vi "Global_SEN_Data Out.vi"() -> ()   [LabVIEW 2020, in "GameController_SEN.lvlib"]
uses:
  GameController_SEN.lvlib
panel:
  in  "SEN_GameController_POVs 1":i16[](array[numeric])
  in  "SEN_GameController_Buttons 1":bool[](array[boolean])
  in  "SEN_GameController_Axes 1":dbl[](array[numeric])
  in  "SEN_GameController_POVs 0":i16[](array[numeric])
  in  "SEN_GameController_Buttons 0":bool[](array[boolean])
  in  "SEN_GameController_Axes 0":dbl[](array[numeric])
  in  "SEN_GameController_CycleTime(S)":dbl
  # "The Names of the Data items in the Global Variable MUST describe who the Single Writer is\nFor Sensor Globals the the naming convention is\n   \nSEN_Lib Name_Data Name\n\nExamples:\nSEN_Gyro_Angle\nSEN_Sonar_Distance"
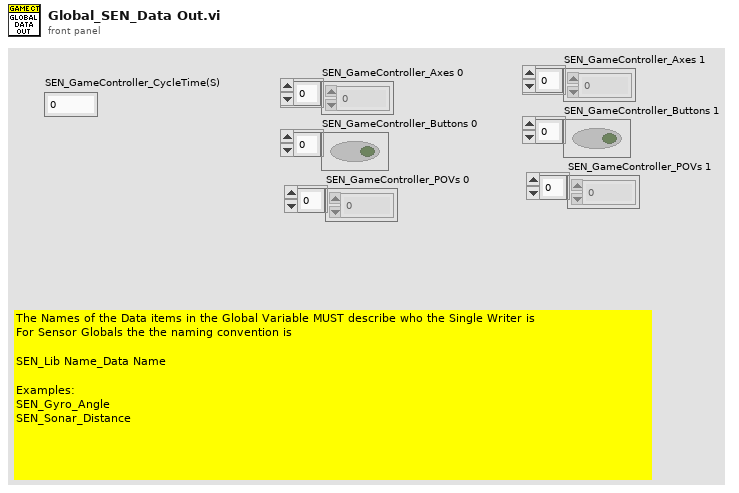
[diagram p1: front panel]
diagram:
